vi "DrawPolygon2D.vi"(1 "Polygon":T1) -> (0 "XYPlot":cluster{dbl[], dbl[]})   [LabVIEW 2017]
uses:
  TypeDefs/Polygon2D.ctl
  TypeDefs/Point2D.ctl
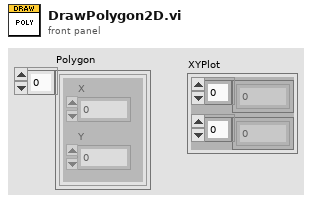
[diagram p1: front panel]
types:
  T1 = typedef "Polygon2D.ctl" = T2[]
  T2 = typedef "Point2D.ctl" = cluster{"X":dbl, "Y":dbl}
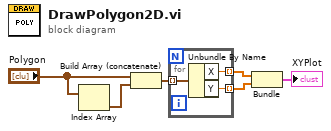
[diagram p0: block diagram]
diagram:
  n1 = Index Array(array="Polygon") -> (element=w3:T2)  [unwired: 1 in]
  n2 = Build Array (concatenate)("Polygon", w3) -> (w4:T1)
  n3 = for {
    tunnel: w4 -> [w9] mode=indexing
    tunnel: [w8] -> w5 mode=indexing
    tunnel: [w7] -> w6 mode=indexing
    n4 = Unbundle By Name(w9) -> ("X"=w8:dbl, "Y"=w7:dbl)
  }
  n5 = Bundle(w5, w6) -> (→"XYPlot":cluster{dbl[], dbl[]})  [unwired: 1 in]
